vi "controlCalculations.vi"(11 "Controller In":refnum<class "Controller.lvclass">) -> (3 "Controller.lvclass":refnum<class "Controller.lvclass">)   [LabVIEW 2016, in "Controller.lvclass"]
uses:
  Controller.lvclass
  Controller.lvclass/Controller.ctl
  View/View.lvclass/View.ctl
  Model/Model.lvclass/Model.ctl
  View/View.lvclass
  Model/Model.lvclass
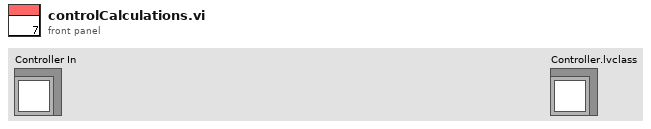
[diagram p1: front panel]
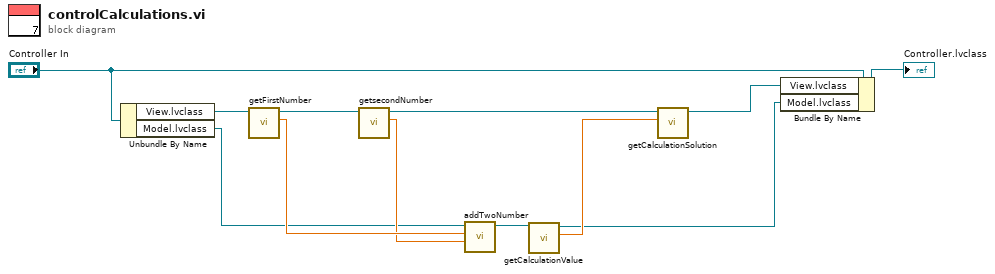
[diagram p0: block diagram]
diagram:
  n1 = Unbundle By Name("Controller In") -> ("View.lvclass"=w12:refnum<class "View.lvclass">, "Model.lvclass"=w8:refnum<class "Model.lvclass">)
  n2 = call "getFirstNumber.vi"("View in"=w12) -> ("firstNumber"=w10:dbl, "View out"=w11:refnum<class "View.lvclass">)  [unwired: 8 in, 1 out]
  n3 = call "getsecondNumber.vi"("View in"=w11) -> ("secondNumber"=w9:dbl, "View out"=w6:refnum<class "View.lvclass">)  [unwired: 8 in, 1 out]
  n4 = call "addTwoNumber.vi"("secondNumber"=w9, "firstNumber"=w10, "Model In"=w8) -> ("Model out"=w7:refnum<class "Model.lvclass">)  [unwired: 8 in]
  n5 = call "getCalculationValue.vi"("Model in"=w7) -> ("calculationValue"=w5:dbl, "Model out"=w1:refnum<class "Model.lvclass">)  [unwired: 8 in, 1 out]
  n6 = call "getCalculationSolution.vi"("calculationResult"=w5, "View.lvclass"=w6) -> ("View out"=w2:refnum<class "View.lvclass">)  [unwired: 9 in]
  n7 = Bundle By Name(cluster="Controller In", "View.lvclass"=w2, "Model.lvclass"=w1) -> (→"Controller.lvclass":refnum<class "Controller.lvclass">)
